vi "Sequence.ConvertColumnHeadersToChannels.vi"(8 "error in (no error)":errorcluster, 9 "Aliases.Outputs":T1[](array[typedef]), 10 "UI.Sequence#ofColumns":i32, 11 "UI.SequenceRef":refnum<vi>) -> (0 "error out":errorcluster, 1 "Warning":string, 3 "Output Channels":T1[](array[typedef]))   [LabVIEW 2013, in "Simple Sequence Editor.lvlib"]
uses:
  Simple Sequence Editor.lvlib
  Types/ChannelProperties.ctl
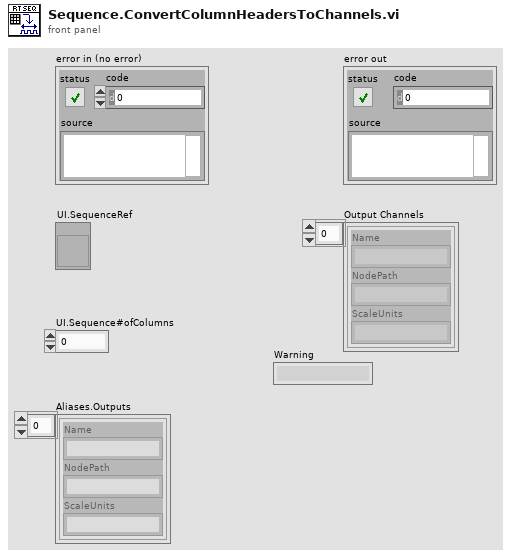
[diagram p1: front panel]
types:
  T1 = typedef "Simple Sequence Editor.lvlib/ChannelProperties.ctl" = cluster{"Name":string, "NodePath":string, "ScaleUnits":string}
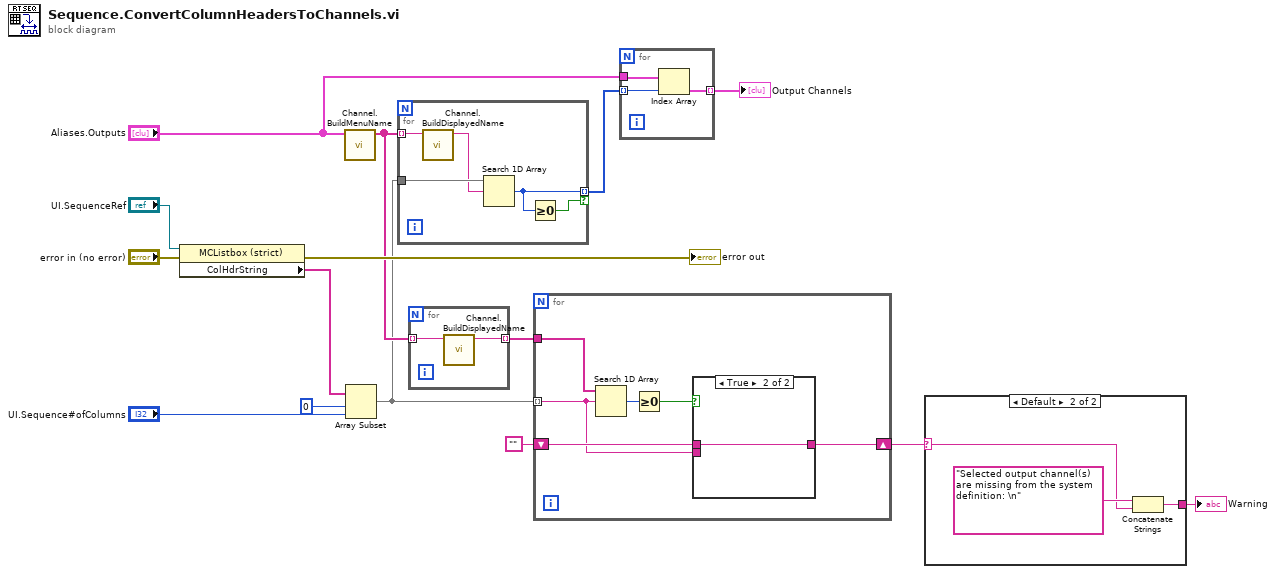
[diagram p0: block diagram]
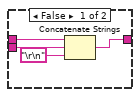
[diagram p3: hidden frame]
diagram:
  n1 = property class="MCListbox (strict)"(reference="UI.SequenceRef", error in="error in (no error)") -> (error out=→"error out":errorcluster, "ColHdrString"=w2:string[])  [unwired: 1 out]
  n2 = call "Channel.BuildMenuName.vi"("Aliases"="Aliases.Outputs") -> ("Aliases Array"=w7:string[])  [unwired: 10 in]
  n3 = Array Subset(array=w2, index=0, length="UI.Sequence#ofColumns") -> (w1:string[])
  n4 = for {
    tunnel: w7 -> [w18] mode=indexing
    tunnel: w1 -> [w20]
    tunnel: [w17] -> w12 mode=indexing if=w16
    n5 = call "Channel.BuildDisplayedName.vi"("Path"=w18) -> ("Formated Path"=w19:string)  [unwired: 10 in]
    n6 = Search 1D Array(1D array=w20, element=w19) -> (index of element=w17:i32)  [unwired: 1 in]
    n7 = Greater Or Equal To 0?(x=w17) -> (x >= 0?=w16:bool)
  }
  n8 = for {
    tunnel: w7 -> [w22] mode=indexing
    tunnel: [w21] -> w6 mode=indexing
    n9 = call "Channel.BuildDisplayedName.vi"("Path"=w22) -> ("Formated Path"=w21:string)  [unwired: 10 in]
  }
  n10 = for {
    tunnel: w6 -> [w27]
    tunnel: w1 -> [w24] mode=indexing
    shift-right: [w25] -> w4
    shift-left: "" -> [w26]
    n11 = Search 1D Array(1D array=w27, element=w24) -> (index of element=w28:i32)  [unwired: 1 in]
    n12 = Greater Or Equal To 0?(x=w28) -> (x >= 0?=w23:bool)
    n13 = case shown="True" w23 {
      tunnel: w26 -> [w31 w33]
      tunnel: [w30 w33] -> w25
      tunnel: w24 -> [w29 _]
      frame False {
        n14 = Concatenate Strings(w31, w29, "\r\n") -> (w30:string)
      }
      frame True {
      }
    }
  }
  n15 = for {
    tunnel: w12 -> [w35] mode=indexing
    tunnel: "Aliases.Outputs" -> [w36]
    tunnel: [w34] -> w11 mode=indexing
    n16 = Index Array(array=w36, index=w35) -> (element=w34:T1)
  }
  "Output Channels" <- w11
  n17 = case shown="Default" w4 {
    selector: w4 -> [w37 w38]
    tunnel: [w37 w39] -> w3
    frame "" {
    }
    frame Default {
      n18 = Concatenate Strings("Selected output channel(s) are missing from the system definition: \n" ("format string"), w38) -> (w39:string)
    }
  }
  "Warning" <- w3
